vi "write-RAW-DATA-SD.vi"(1 "error in (no error)":errorcluster, 2 "Text":string, 3 "File":path) -> (0 "error out":errorcluster)   [LabVIEW 2015]
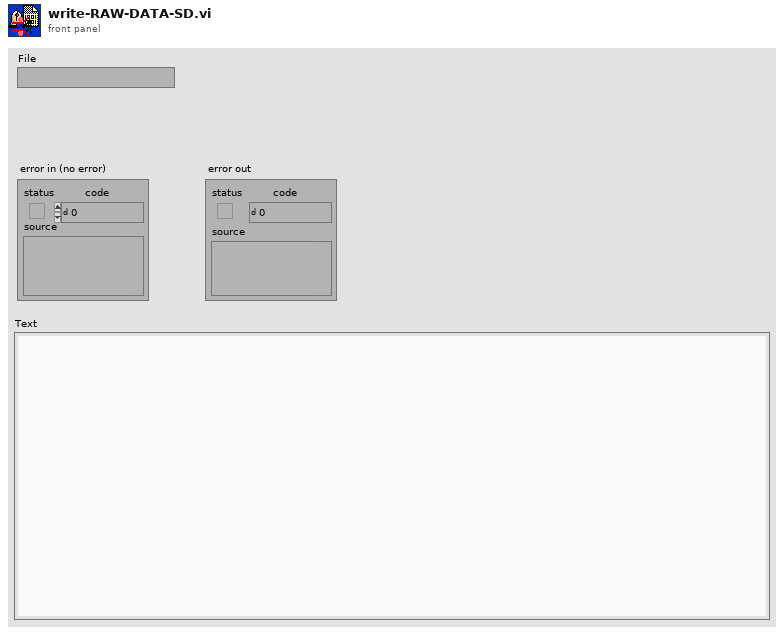
[diagram p1: front panel]
types:
  T1 = enum16{"open", "replace", "create", "open or create", "replace or create", "replace or create with confirmation"}
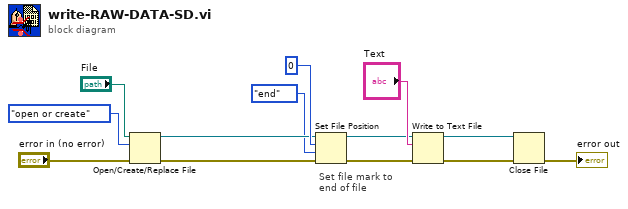
[diagram p0: block diagram]
diagram:
  # "Set file mark to\nend of file"
  n1 = Open/Create/Replace File(file path (use dialog)="File", error in="error in (no error)", operation (0:open)=T1."open or create") -> (refnum out=w9:refnum<file>, error out=w10:errorcluster)  [unwired: 3 in, 1 out]
  n2 = Set File Position(offset (in bytes) (0)=i64 0, refnum=w9, from (0:start)=enum16{"start", "end", "current"}."end", error in=w10) -> (refnum out=w4:refnum<file>, error out=w3:errorcluster)
  n3 = Write to Text File(file (use dialog)=w4, text="Text", error in=w3) -> (refnum out=w7:refnum<file>, error out=w6:errorcluster)  [unwired: 1 in, 1 out]
  n4 = Close File(refnum=w7, error in=w6) -> (error out=→"error out":errorcluster)  [unwired: 1 out]
